vi "Configure Frequency.vi"(0 "VISA resource name":refnum<visa-resource-name>, 1 "Enable Auto Range (T:Enable)":bool=TRUE, 4 "Manual Range (0 V)":dbl format="%#_6p", 5 "error in (no error)":errorcluster, 8 "Sampling Rate (4: SLOW)":u16(ring)=4 format="%.0g" items=["FAST"=1, "MED"=3, "SLOW"=4], 12 "Digits (5: 5 1/2)":u16(ring)=5 format="%.0g" items=["3 1/2 Digits"=3, "4 1/2 Digits"=4, "5 1/2 Digits"=5]) -> (14 "VISA resource name out":refnum<visa-resource-name>, 19 "error out":errorcluster)   [LabVIEW 2017, in "ADCMT7451_ADC.lvlib"]
doc: "Configures the measurement type, resolution, and range on the instrument."
uses:
  ADCMT7451_ADC.lvlib
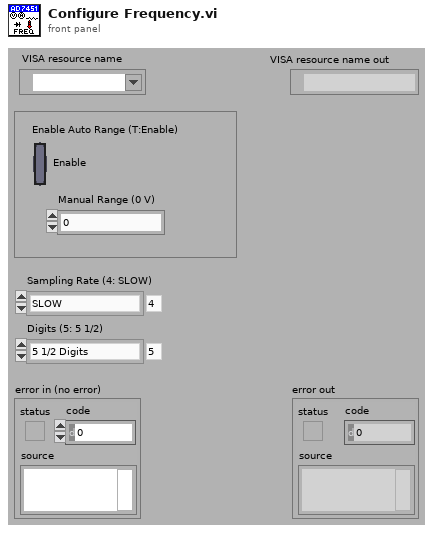
[diagram p1: front panel]
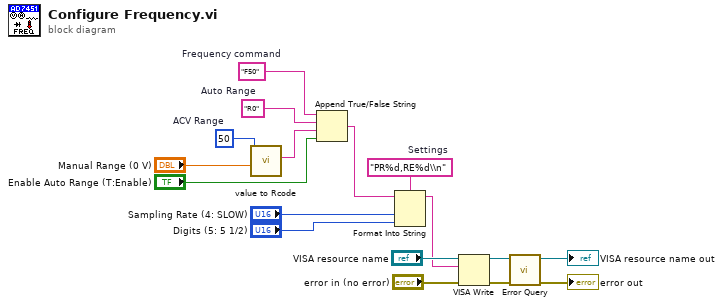
[diagram p0: block diagram]
diagram:
  w5 = "PR%d,RE%d\\n"  # Settings
  w8 = "F50"  # Frequency command
  w10 = 50  # ACV Range
  w11 = "R0"  # Auto Range
  n1 = call "value to Rcode.vi"("Manual Range (0)"="Manual Range (0 V)", "Function (1: DC Volts)"=w10) -> ("Range Set Code"=w9:string)  [unwired: 9 in]
  n2 = Append True/False String(1:"Enable Auto Range (T:Enable)", 2:w9, 3:w11, 4:w8) -> (0:w4:string)
  n3 = Format Into String(format string=w5, initial string=w4, "Sampling Rate (4: SLOW)", "Digits (5: 5 1/2)") -> (resulting string=w1:string)  [unwired: 1 in, 1 out]
  n4 = VISA Write(VISA resource name="VISA resource name", write buffer=w1, error in (no error)="error in (no error)") -> (VISA resource name out=w13:refnum<visa-resource-name>, error out=w12:errorcluster)  [unwired: 1 out]
  n5 = call "Error Query.vi"("error in (no error)"=w12, "VISA resource name"=w13) -> ("error out"=→"error out":errorcluster, "VISA resource name out"=→"VISA resource name out":refnum<visa-resource-name>)  [unwired: 6 in, 2 out]
